vi "Initialize.vi"(8 "error in (no error)":errorcluster, 9 "Camera Type":T1, 10 "DAQ Configuration":T2={"Shutters"=[], "fluidics trigger line"="Dev1/port1/line1", "camera trigger line"="", "COM Port"="COM3", "Device type"=enum."NI DAQ"}, 11 "Synchronization Device in":refnum<class "Arduino DAQ.lvclass">) -> (0 "error out":errorcluster, 3 "Synchronization Device out":refnum<class "Arduino DAQ.lvclass">, 4 "Trigger Jitter (ms)":dbl)   [LabVIEW 2023, in "Arduino DAQ.lvlib" / "Arduino DAQ.lvclass"]
uses:
  Arduino DAQ.lvclass
  Resources/Type Defs/DAQ Configuration.ctl
  Resources/Type Defs/Shutter Configuration.ctl
  Resources/Type Defs/Sync Device Type.ctl
  Arduino DAQ.lvclass/Arduino DAQ.ctl
  <vilib>/Instr/_visa.llb/VISA Configure Serial Port (Instr).vi
  Resources/Type Defs/Camera Type.ctl
panel:
  out "Startup Message":string
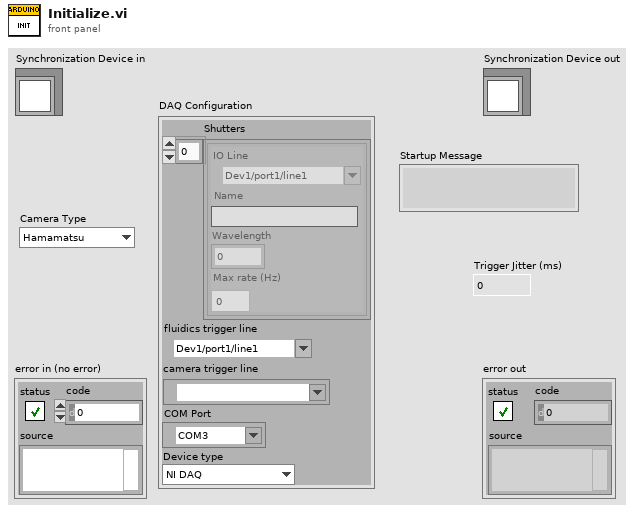
[diagram p1: front panel]
types:
  T1 = typedef "Camera Type.ctl" = enum16{"Hamamatsu", "Andor", "Photometrics"}
  T2 = typedef "DAQ Configuration.ctl" = cluster{"Shutters":T3[], "fluidics trigger line":tag, "camera trigger line":tag, "COM Port":refnum<visa-resource-name>, "Device type":T4}
  T3 = typedef "Shutter Configuration.ctl" = cluster{"IO Line":tag, "Name":string, "Wavelength":u16, "Max rate (Hz)":dbl}
  T4 = typedef "Sync Device Type.ctl" = enum16{"Disabled", "NI DAQ", "Arduino DAQ", "Microsync"}
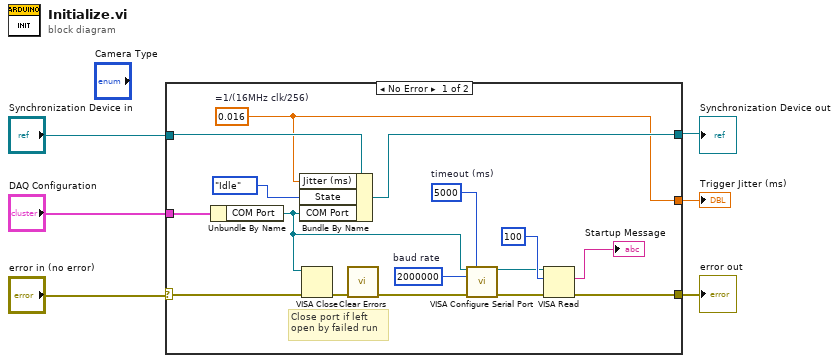
[diagram p0: block diagram]
diagram:
  n1 = case shown="No Error" "error in (no error)" {
    selector: "error in (no error)" -> [w12 w24]
    tunnel: [w8 w24] -> w5
    tunnel: [w15 w23] -> w3
    tunnel: "Synchronization Device in" -> [w16 w23]
    tunnel: "DAQ Configuration" -> [w14 _]
    tunnel: [w7 _] -> w1
    frame No Error {
      w7 = 0.016  # =1/(16MHz clk/256)
      w21 = u32 5000  # timeout (ms)
      w22 = u32 2000000  # baud rate
      # "Close port if left\nopen by failed run"
      n2 = Unbundle By Name(w14) -> ("COM Port"=w10:refnum<visa-resource-name>)
      n3 = Bundle By Name(cluster=w16, "Jitter (ms)"=w7, "State"=enum16{"Idle", "Manual", "Stream"}."Idle", "COM Port"=w10) -> (w15:refnum<class "Arduino DAQ.lvclass">)
      n4 = VISA Close(VISA resource name=w10, error in (no error)=w12) -> (error out=w13:errorcluster)
      n5 = call <vilib>:"Clear Errors.vi"("error in (no error)"=w13) -> ("error out"=w11:errorcluster)  [unwired: 5 in, 1 out]
      n6 = call-poly "VISA Configure Serial Port"("VISA resource name"=w10, "timeout (10sec)"=w21, "baud rate (9600)"=w22, "error in (no error)"=w11) -> ("VISA resource name out"=w17:refnum<visa-resource-name>, "error out"=w18:errorcluster)  [unwired: 10 in]
      n7 = VISA Read(VISA resource name=w17, byte count=u32 100, error in (no error)=w18) -> (read buffer=→"Startup Message":string, error out=w8:errorcluster)  [unwired: 2 out]
    }
    frame Error {
    }
  }
  "error out" <- w5
  "Synchronization Device out" <- w3
  "Trigger Jitter (ms)" <- w1
